vi "dfd_Super Narrowband Filter Design Call New Method.vi"(5 "M":i32, 6 "ripple specs":T6, 7 "new filter type":T7(ring), 8 "error in (no error)":errorcluster, 10 "fstop":dbl, 11 "fpass":dbl) -> (0 "error out":errorcluster, 3 "multirate filters out":T1[](array[typedef]) {"mMRate_SumWl" min=1 max=32 step=1; "mMRate_InputIwl" min=1 max=32 step=1; "mMRate_GainWl" min=1 max=32 step=1; "mMRate_OutputWl" min=1 max=32 step=1; "mMRate_InputWl" min=1 max=32 step=1; "mMRate_CoefWl" min=1 max=32 step=1; "mMRate_Mode" items=["Default"=-1, "No Rate Change"=0, "Interpolation"=1, "Decimation"=2, "Interpolated"=3, "Rational"=4]})   [LabVIEW 2017, in "NI_DigFilter_Process.lvlib"]
uses:
  <vilib>/addons/Digital Filter Design/NI_DigFilter_Process.lvlib
  <vilib>/addons/Digital Filter Design/_Objects.llb/DFD Filter Ripple Specification (Design).ctl
  <vilib>/addons/Digital Filter Design/_Objects.llb/DFD Multirate Filter Obj.ctl
  <vilib>/addons/Digital Filter Design/_Objects.llb/DFD Multirate Mode.ctl
  <vilib>/addons/Digital Filter Design/_Objects.llb/DFD Coef Norm Type.ctl
  <vilib>/addons/Digital Filter Design/_Objects.llb/DFD Round-off Mode.ctl
  <vilib>/addons/Digital Filter Design/_Objects.llb/DFD FXP MRate Multiply Mode.ctl
  <vilib>/addons/Digital Filter Design/_Objects.llb/DFD Filter Frequence Specification (Design).ctl
  <vilib>/addons/Digital Filter Design/NI_DigFilterLicensed.lvlib
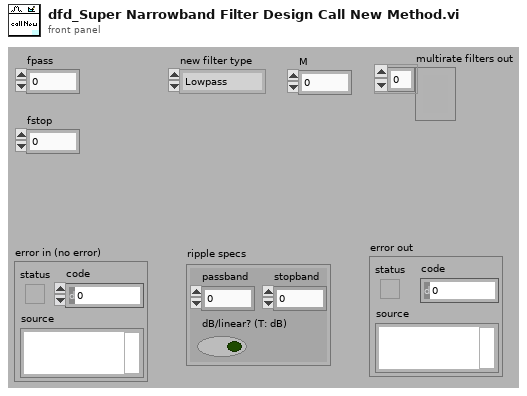
[diagram p1: front panel]
types:
  T1 = typedef "NI_DigFilterLicensed.lvlib/DFD Multirate Filter Obj.ctl" = cluster{"mMRate_Structure":enum16{"CIC", "FIR", "IIR", "Lattice"}, "mMRate_Mode":T2, "mMRate_Factor":i32, "mMRate_FIRParams":cluster{"mMRate_FIR_H":dbl[], "mMRate_FIR_IsNyquist?":bool, "mMRate_FIR_IsSymmetric?":bool}, "mMRate_CICParams":cluster{"mMRate_CIC_#Stage":i32, "mMRate_CIC_Lag":i32, "mMRate_CIC_Type":enum16{"Lowpass", "Highpass"}}, "mMRate_Order":i32, "mMRate_Version":string, "mMRate_Comments":string, "mMRate_RationalFactor":cluster{"mMRate_L":i32, "mMRate_M":i32}, "mMRate_Fs":dbl, "mMRate_Quantized?":bool, "mMRate_QFilterGain":dbl, "mMRate_CoefWl":i16, "mMRate_Scaling":cluster{"mMRate_ScaleByPowerOf2?":bool, "mMRate_ScaleType":T3}, "mMRate_InputWl":i16, "mMRate_OutputWl":i16, "mMRate_OutputMode":T4, "mMRate_MultMode":T5, "mMRate_BitPruning":bool, "mMRate_GainWl":i16, "mMRate_OutputFwl":i16, "mMRate_SumIwl":i16, "mMRate_InputIwl ":i16, "mMRate_SumWl":i16, "mMRate_CoefIwl":i16}
  T2 = typedef "NI_DigFilterLicensed.lvlib/DFD Multirate Mode.ctl" = i16
  T3 = typedef "NI_DigFilterLicensed.lvlib/DFD Coef Norm Type.ctl" = enum16{"No Norm", "Time Domain 1-Norm", "Time Domain 2-Norm", "Time Domain Inf-Norm"}
  T4 = typedef "NI_DigFilterLicensed.lvlib/DFD Round-off Mode.ctl" = enum16{"Nearest", "Truncation"}
  T5 = typedef "NI_DigFilterLicensed.lvlib/DFD FXP MRate Multiply Mode.ctl" = enum16{"Truncated", "Full"}
  T6 = typedef "NI_DigFilterLicensed.lvlib/DFD Filter Ripple Specification (Design).ctl" = cluster{"passband":dbl, "stopband":dbl, "dB/linear? (T: dB)":bool}
  T7 = enum32{"Lowpass", "Highpass", "Bandpass", "Bandstop", "Wideband-Lowpass", "Wideband-Highpass"}
  T8 = typedef "NI_DigFilterLicensed.lvlib/DFD Filter Frequence Specification (Design).ctl" = cluster{"fpass 1":dbl, "fstop 1":dbl, "fpass 2 ":dbl, "fstop 2":dbl}
  T9 = typedef "NI_DigFilterLicensed.lvlib/DFD Adv Band Spec.ctl" = cluster{"band specification":cluster{"freq":dbl, "amplitude":dbl, "weight":dbl}[], "ripple constraint":dbl}
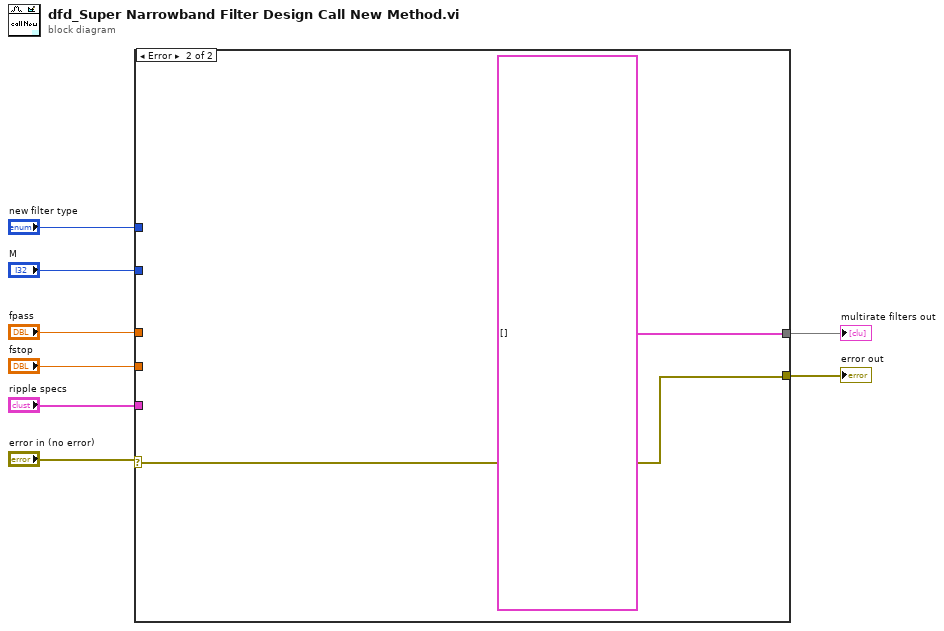
[diagram p0: block diagram]
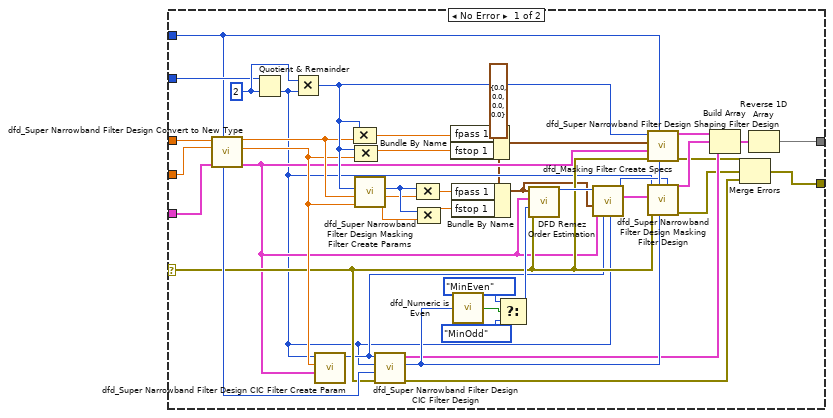
[diagram p2: hidden frame]
diagram:
  n1 = case shown="Error" "error in (no error)" {
    selector: "error in (no error)" -> [w19 w50]
    tunnel: "new filter type" -> [w31 _]
    tunnel: "M" -> [w44 _]
    tunnel: "fpass" -> [w48 _]
    tunnel: "fstop" -> [w47 _]
    tunnel: "ripple specs" -> [w46 _]
    tunnel: [w22 w50] -> w2
    tunnel: [w11 T1[] [] ("Array")] -> w1
    frame No Error {
      w14 = T8 {"fpass 1"=0.0, "fstop 1"=0.0, "fpass 2 "=0.0, "fstop 2"=0.0} ("Shaping freq specs [Hz]")
      w45 = 2 ("y")
      n2 = call <vilib>:"dfd_Super Narrowband Filter Design Convert to New Type.vi"("new filter type"=w31, "ripple specs"=w46, "fstop"=w47, "fpass"=w48) -> ("ripple specs out"=w18:T6, "fstop out"=w32:dbl, "fpass out"=w39:dbl)  [unwired: 1 in, 4 out]
      n3 = Quotient & Remainder(x=w44, y=w45) -> (floor(x/y)=w16:i32)  [unwired: 1 out]
      n4 = Multiply(x=w45, y=w16) -> (x*y=w40:i32)
      n5 = call <vilib>:"dfd_Super Narrowband Filter Design CIC Filter Create Param.vi"("ripple spec"=w18, "shaping original fstop"=w32, "CIC factor"=w16) -> ("CIC stage"=w17:i32)  [unwired: 8 out]
      n6 = Compound Arithmetic op=MULTIPLY(w40, w39) -> (w43:dbl)
      n7 = Compound Arithmetic op=MULTIPLY(w40, w32) -> (w42:dbl)
      n8 = call <vilib>:"dfd_Super Narrowband Filter Design Masking Filter Create Params.vi"("fstop"=w32, "fpass"=w39, "shaping M"=w40) -> ("masking original fstop"=w10:dbl, "masking original fpass"=w37:dbl, "masking N"=w38:i32)  [unwired: 1 in, 5 out]
      n9 = call <vilib>:"dfd_Super Narrowband Filter Design CIC Filter Design.vi"("error in (no error)"=w19, "filter type"=w31, "N"=w16, "CIC stage"=w17) -> ("error out"=w23:errorcluster, "order"=w27:i32, "CIC filter out"=w26:T1)  [unwired: 5 out]
      n10 = Compound Arithmetic op=MULTIPLY(w38, w37) -> (w13:dbl)
      n11 = Compound Arithmetic op=MULTIPLY(w38, w10) -> (w12:dbl)
      n12 = Bundle By Name(cluster=w14, "fpass 1"=w43, "fstop 1"=w42) -> (w41:T8)
      n13 = Bundle By Name(cluster=w14, "fpass 1"=w13, "fstop 1"=w12) -> (w9:T8)
      n14 = call <vilib>:"dfd_Numeric is Even.vi"("N"=w27) -> ("even ?"=w36:bool)
      n15 = Select(t=enum16{"MinNum", "MinEven", "MinOdd"}."MinEven" ("order option"), s=w36, f=enum16{"MinNum", "MinEven", "MinOdd"}."MinOdd" ("order option")) -> (s? t:f=w33:enum16{"MinNum", "MinEven", "MinOdd"})
      n16 = call <vilib>:"DFD Remez Order Estimation.vi"("error in (no error)"=w19, "order option"=w33, "ripple specs"=w18, "freq specs [Hz]"=w9) -> ("estimated order"=w20:i32)  [unwired: 2 in, 5 out]
      n17 = call <vilib>:"dfd_Masking Filter Create Specs.vi"("CIC factor"=w16, "CIC stage"=w17, "ripple specs"=w18, "masking freq specs [Hz]"=w9, "masking order"=w20) -> ("Masking band parameters"=w15:T9[], "dup masking order"=w21:i32)  [unwired: 2 in, 3 out]
      n18 = call <vilib>:"dfd_Super Narrowband Filter Design Shaping Filter Design.vi"("filter type"=w31, "error in (no error)"=w19, "Shaping ripple specs"=w18, "Shaping freq specs [Hz]"=w41, "M"=w40) -> ("error out"=w25:errorcluster, "Shaping filter"=w29:T1)  [unwired: 5 out]
      n19 = call <vilib>:"dfd_Super Narrowband Filter Design Masking Filter Design.vi"("masking order"=w21, "CIC order"=w27, "filter type"=w31, "error in (no error)"=w19, "Masking band parameters"=w15, "N"=w16) -> ("error out"=w24:errorcluster, "multirate filter out"=w28:T1)  [unwired: 4 out]
      n20 = Build Array(w29, w28, w26) -> (w30:T1[])
      n21 = Merge Errors(w25, w24, w23) -> (w22:errorcluster)
      n22 = Reverse 1D Array(array=w30) -> (reversed array=w11:T1[])
    }
    frame Error {
    }
  }
  "multirate filters out" <- w1
  "error out" <- w2
